vi "xc_umn_XPS_and_LockinControl_GPIB.vi"() -> ()   [LabVIEW 2013]
uses:
  <vilib>/Analysis/baseanly.llb/Mean (DBL).vi
  <vilib>/Utility/file.llb/Write To Spreadsheet File (DBL).vi
  <vilib>/Analysis/NI_AALBase.lvlib
panel:
  in  "?":string
  in  "?":T1(tab)
  out "Waveform Graph":dbl[](graph)=[0.0, -0.00745064, -0.0298025, -0.0149013, -0.00745064, 0.0, 0.00745064, 0.022351899999999997, 0.0149013, 0.00745064, -0.0298025, 0.0149013, 0.0, -0.0447037, -0.00745064, -0.00745064, 0.022351899999999997, 0.0, 0.0, -0.00745064, 0.037253100000000004, -0.00745064, -0.0298025, 0.0, -0.0149013, 0.0, 0.0, -0.0670557, -0.0149013, 0.0149013, 0.0149013, 0.0, 0.0, 0.0149013, 0.0, 0.0298025, -0.0447037, 0.00745064, -0.037253100000000004, -0.0149013, 0.00745064, 0.037253100000000004, 0.0149013, 0.0, -0.0298025, -0.0149013, 0.00745064, 0.0, -0.0447037, 0.00745064, 0.0149013, 0.022351899999999997, 0.0, -0.022351899999999997, 0.0, 0.037253100000000004, -0.0298025, -0.037253100000000004, -0.00745064, 0.0, -0.00745064, 0.0298025, 0.0149013, 0.0, -0.0298025, 0.0149013, -0.0298025, -0.0298025, -0.00745064, -0.0298025, -0.037253100000000004, -0.022351899999999997, 0.0, -0.0298025, -0.037253100000000004, 0.0149013, -0.00745064, -0.0149013, -0.00745064, 0.0, -0.0447037, 0.0149013, 0.0, -0.037253100000000004, -0.0149013, -0.0298025, -0.0447037, -0.022351899999999997, -0.022351899999999997, 0.0149013, -0.022351899999999997, 0.0, -0.022351899999999997, 0.022351899999999997, 0.0, 0.037253100000000004, -0.022351899999999997, 0.022351899999999997, -0.0298025, -0.022351899999999997]
  in  "Start Button":bool
  in  "quit Button":bool
  in  "save":bool
  out "Current Mean":dbl=-0.0275905 format="%#_10g"
  out "Current position":dbl=-9.999556
  in  "Range (in mm)":dbl=1.0
  in  "Increment (in mm)":dbl=0.01
  in  "Averages":u16=1
  in  "Start Position":dbl=-10.0
  in  "move":bool
  out "Compensation":dbl=1000000.0
  in  "Position":dbl
  in  "Left jog":bool
  in  "Jog step size (mm)":dbl=0.01
  in  "Right jog":bool
  out "Stage Position":dbl=1e-06
  in  "Move to Position Button":bool
  in  "Time Constant":u16(ring)=7 items=["10 us", "30 us", "100 us", "300 us", "1 ms", "3 ms", "10 ms", "30 ms", "100 ms", "300 ms", "1 s", "3 s", "10 s", "30 s", "100 s", "300 s", "1 ks", "3 ks", "10 ks", "30 ks"]
  in  "Sensitivity":u16(ring)=9 items=["2 nV/fA", "5 nV/fA", "10 nV/fA", "20 nV/fA", "50 nV/fA", "100 nV/fA", "200 nV/fA", "500 nV/fA", "1 uV/pA", "2 uV/pA", "5 uV/pA", "10 uV/pA", "20 uV/pA", "50 uV/pA", "100 uV/pA", "200 uV/pA", "500 uV/pA", "1 mV/nA", "2 mV/nA", "5 mV/nA", "10 mV/nA", "20 mV/nA", "50 mV/nA", "100 mV/nA", "200 mV/nA", "500 mV/nA", "1 V/uA"]
  in  "Input Configuration":u16(ring) items=["A", "A-B", "1 MOhm", "10 MOhm"]
  out "Sensitivity Compensation":dbl=1000000.0
  in  "Autophase":bool
  out "Scale Unit":string="uV"
  out "Lockin realtime output":dbl(knob)=-0.0275905 scale=-1.0..1.0
  out "Lockin error out":errorcluster={"status"=FALSE, "code"=1073676294, "source"="VISA Read in xc_umn_XPS_and_LockinControl.vi"}
  in  "Lockin error in":errorcluster
  out "Array":dbl[](array[numeric])=[0.0, -0.00745064, -0.0298025, -0.0149013, -0.00745064, 0.0, 0.00745064, 0.022351899999999997, 0.0149013, 0.00745064, -0.0298025, 0.0149013, 0.0, -0.0447037, -0.00745064, -0.00745064, 0.022351899999999997, 0.0, 0.0, -0.00745064, 0.037253100000000004, -0.00745064, -0.0298025, 0.0, -0.0149013, 0.0, 0.0, -0.0670557, -0.0149013, 0.0149013, 0.0149013, 0.0, 0.0, 0.0149013, 0.0, 0.0298025, -0.0447037, 0.00745064, -0.037253100000000004, -0.0149013, 0.00745064, 0.037253100000000004, 0.0149013, 0.0, -0.0298025, -0.0149013, 0.00745064, 0.0, -0.0447037, 0.00745064, 0.0149013, 0.022351899999999997, 0.0, -0.022351899999999997, 0.0, 0.037253100000000004, -0.0298025, -0.037253100000000004, -0.00745064, 0.0, -0.00745064, 0.0298025, 0.0149013, 0.0, -0.0298025, 0.0149013, -0.0298025, -0.0298025, -0.00745064, -0.0298025, -0.037253100000000004, -0.022351899999999997, 0.0, -0.0298025, -0.037253100000000004, 0.0149013, -0.00745064, -0.0149013, -0.00745064, 0.0, -0.0447037, 0.0149013, 0.0, -0.037253100000000004, -0.0149013, -0.0298025, -0.0447037, -0.022351899999999997, -0.022351899999999997, 0.0149013, -0.022351899999999997, 0.0, -0.022351899999999997, 0.022351899999999997, 0.0, 0.037253100000000004, -0.022351899999999997, 0.022351899999999997, -0.0298025, -0.022351899999999997]
  out "Array 2":dbl[](array[numeric])=[-9.989987, -9.979989, -9.969994, -9.959974, -9.949978, -9.939973, -9.929969, -9.919957, -9.909953, -9.899948, -9.889937, -9.879957, -9.869966, -9.85997, -9.849976, -9.839989, -9.82999, -9.819995, -9.809984, -9.799976, -9.789956, -9.77995, -9.769948, -9.759954, -9.749947, -9.739953, -9.729953, -9.719978, -9.70998, -9.699991, -9.689985, -9.679993, -9.669982, -9.660004, -9.649987, -9.639984, -9.629972, -9.619964, -9.609951, -9.59995, -9.58996, -9.579923, -9.569946, -9.559948, -9.549953, -9.539952, -9.529956, -9.519982, -9.509964, -9.499961, -9.489967, -9.479974, -9.469988, -9.459988, -9.449998, -9.439994, -9.429985, -9.419973, -9.409972, -9.399965, -9.389954, -9.37994, -9.369937, -9.35994, -9.349967, -9.339974, -9.330002, -9.319993, -9.309984, -9.299992, -9.289988, -9.279986, -9.269974, -9.259965, -9.249946, -9.239952, -9.229939, -9.219955, -9.209954, -9.199959, -9.189968, -9.179975, -9.169977, -9.159978, -9.149988, -9.139981, -9.129984, -9.119984, -9.109976, -9.099978, -9.089976, -9.07995, -9.069946, -9.059963, -9.049951, -9.039946, -9.029939, -9.019958, -9.009948, -8.999961]
  in  "Lockin GPIB Address":string
  in  "PI Stage Error":errorcluster
  out "PI Stage Error 2":errorcluster
  out "Identification":string="(c)2010 Physik Instrumente(PI) Karlsruhe, C-867.160,0,1.2.0.1"
  # "University of Minnesota Lockin Scan and Optimize\nVersion 2.0\n[XPS Controller; SR830 Lockin; RS232]"
  # "Lockin Output"
  # "Stage Controls"
  # "Lockin Controls"
  # "Lockin Communications"
  # "Stage Communications"
  # "Data Out"
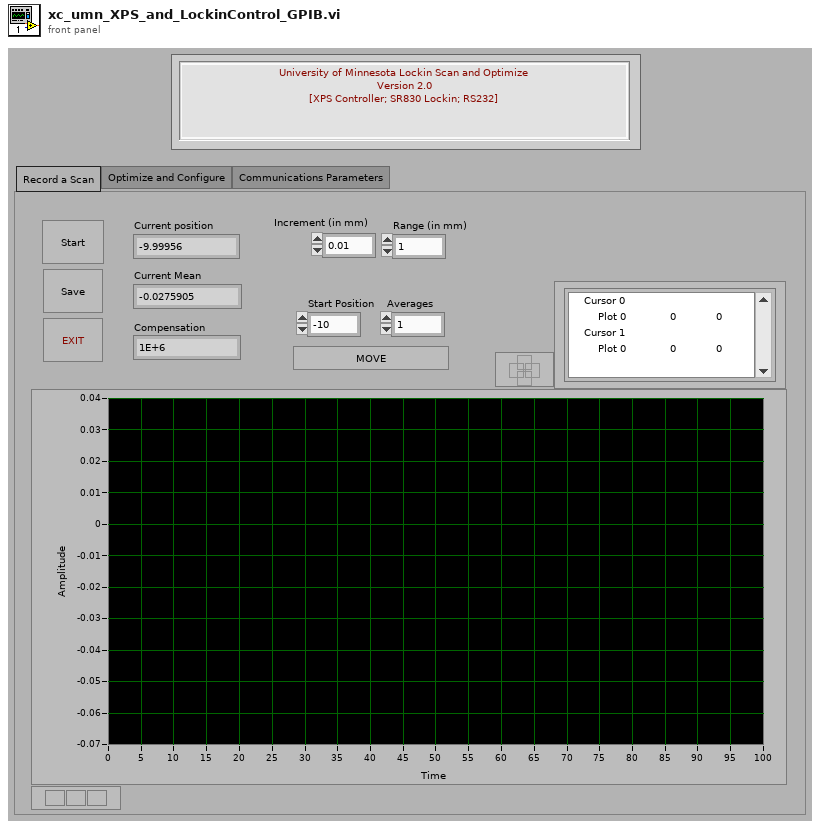
[diagram p1: front panel]
types:
  T1 = enum32{"Record a Scan", "Optimize and Configure", "Communications Parameters"}
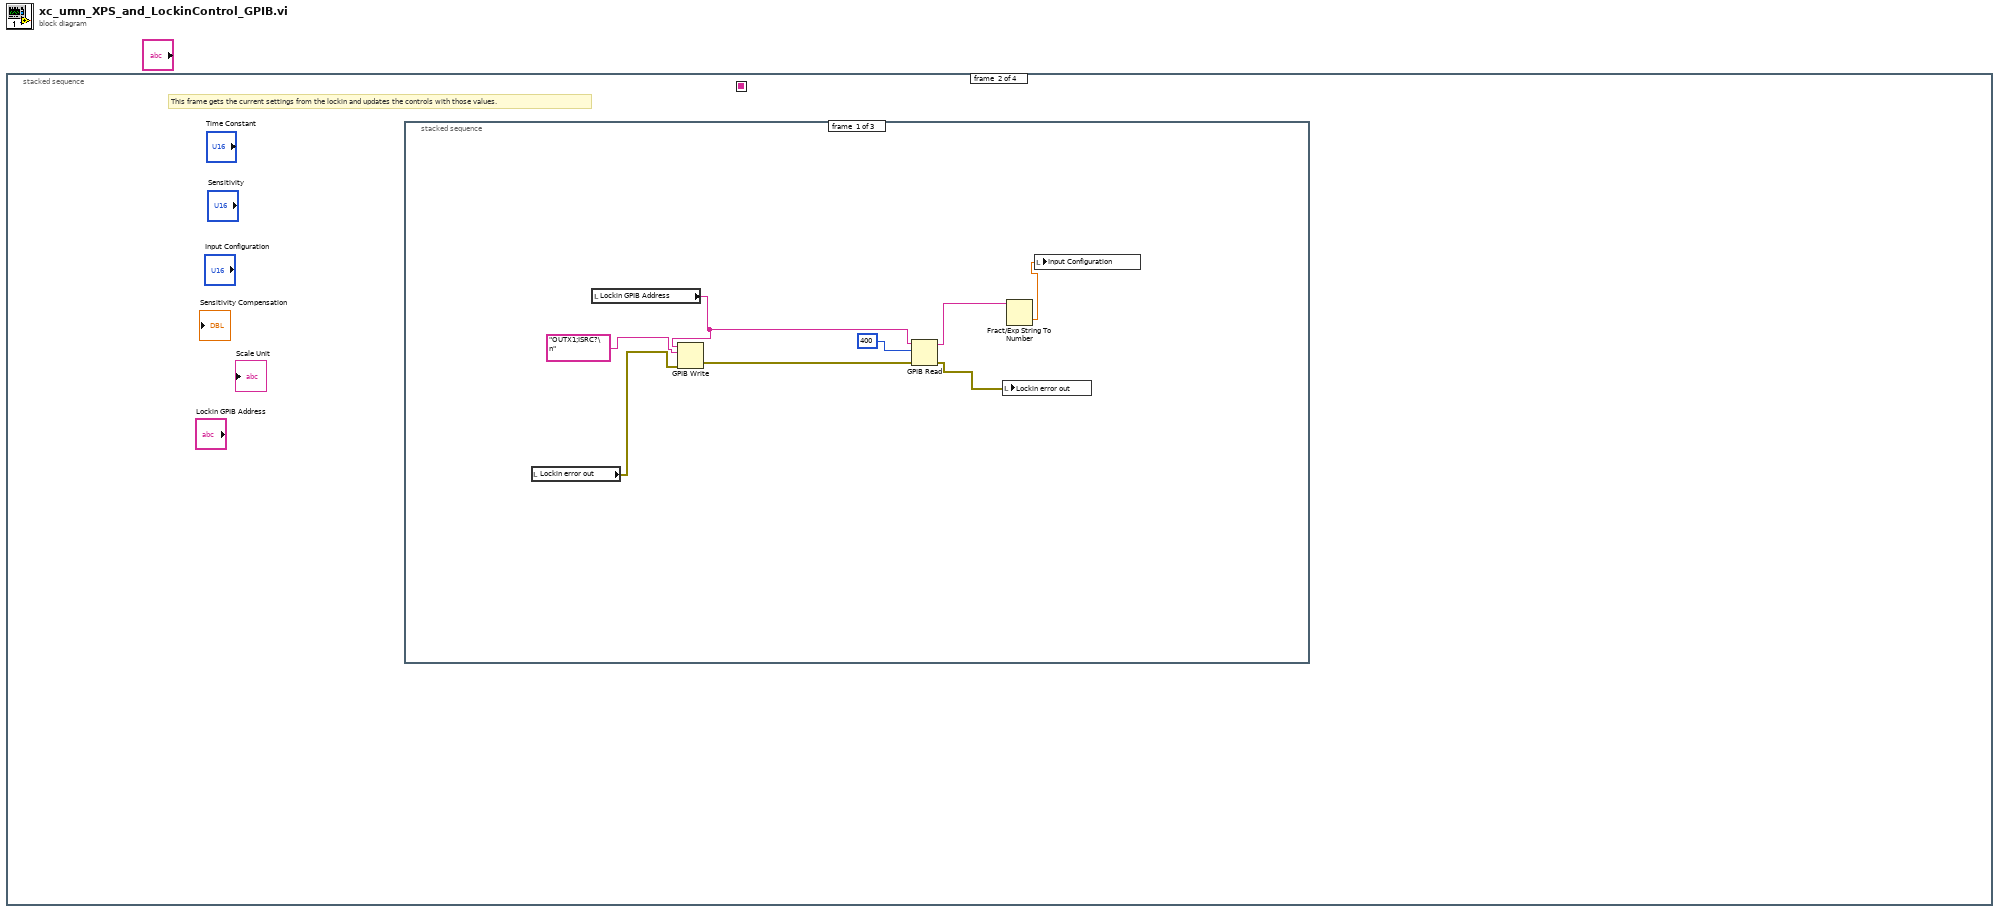
[diagram p0: block diagram]
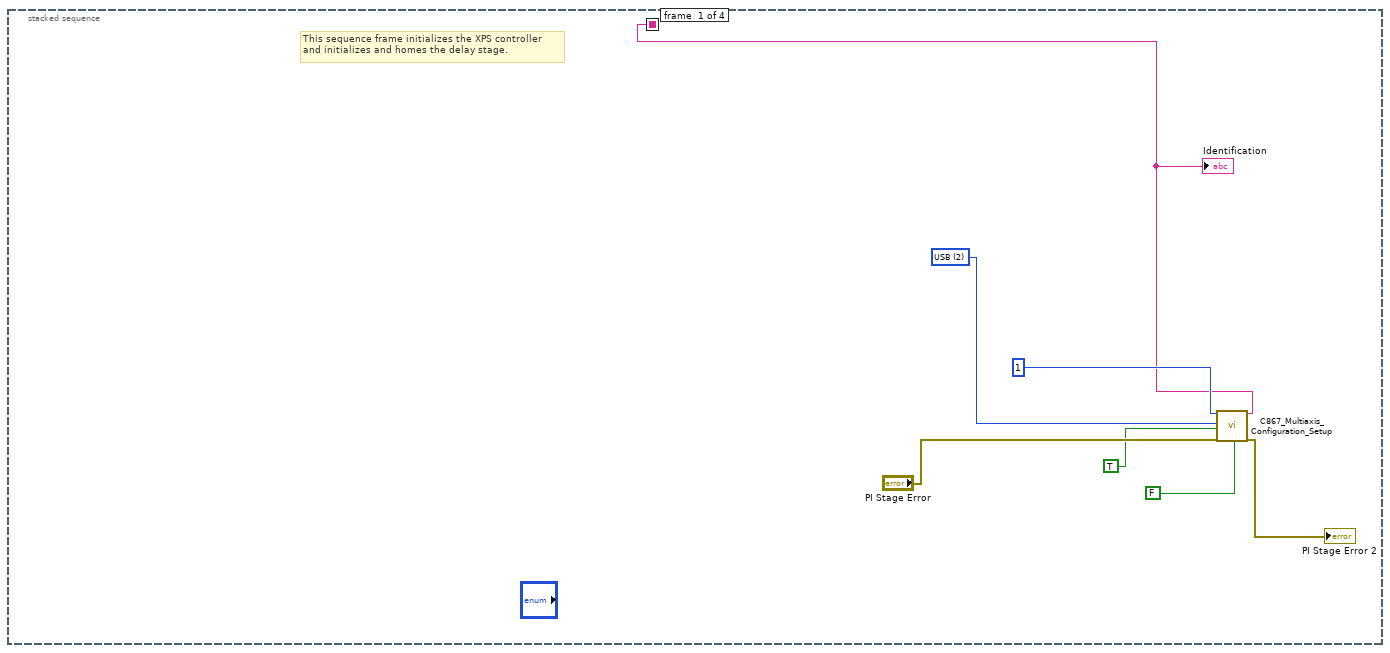
[diagram p2: hidden frame]
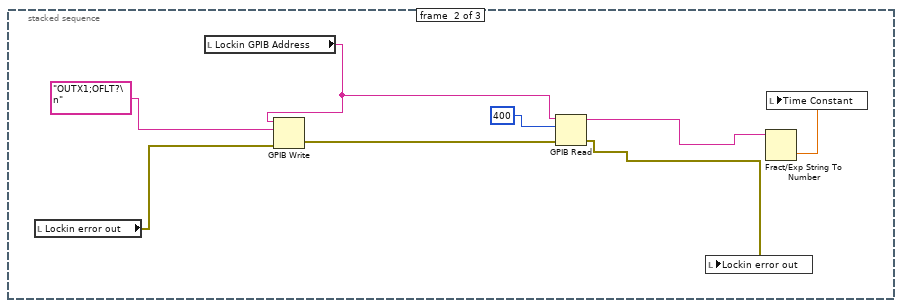
[diagram p3: hidden frame]
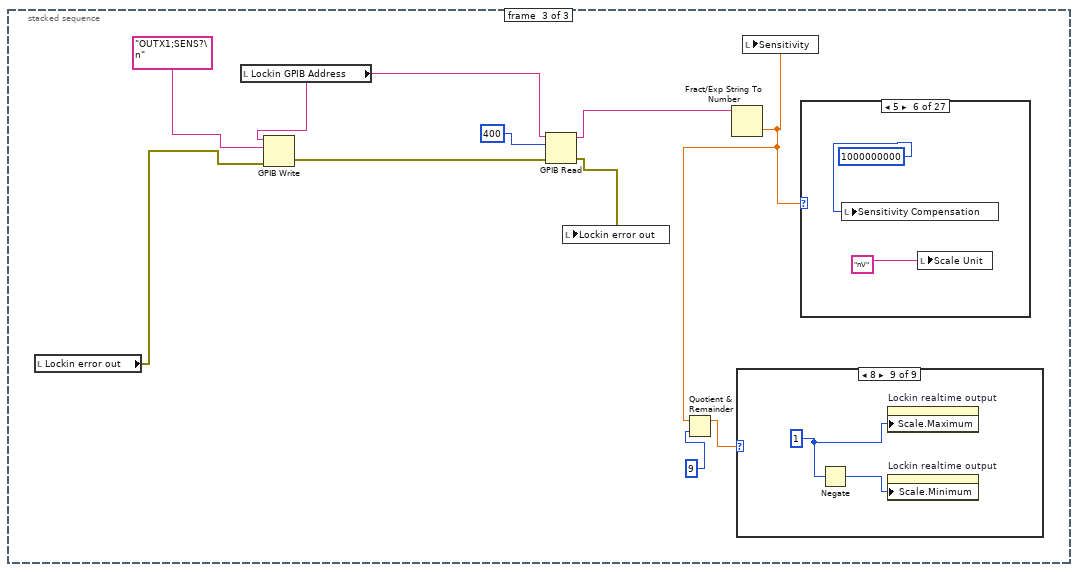
[diagram p4: hidden frame]
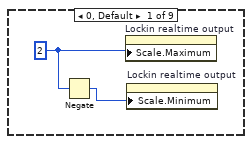
[diagram p5: hidden frame]
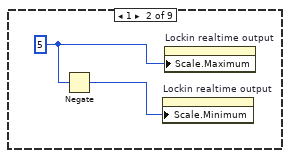
[diagram p6: hidden frame]
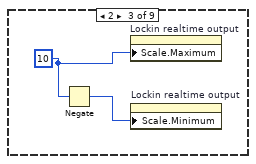
[diagram p7: hidden frame]
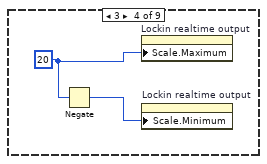
[diagram p8: hidden frame]
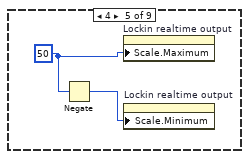
[diagram p9: hidden frame]
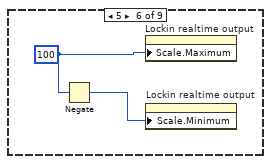
[diagram p10: hidden frame]
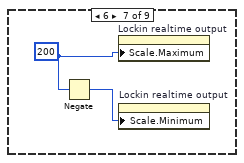
[diagram p11: hidden frame]
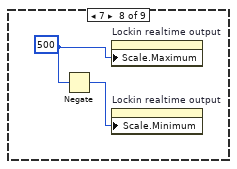
[diagram p12: hidden frame]
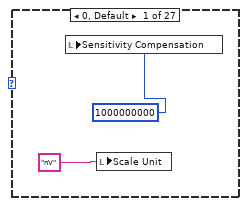
[diagram p13: hidden frame]
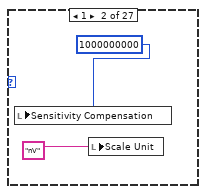
[diagram p14: hidden frame]
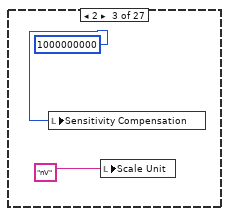
[diagram p15: hidden frame]
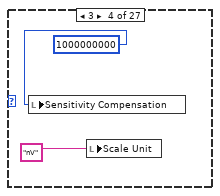
[diagram p16: hidden frame]
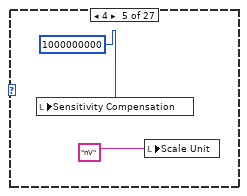
[diagram p17: hidden frame]
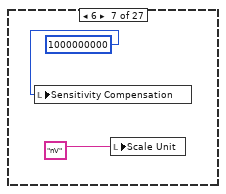
[diagram p18: hidden frame]
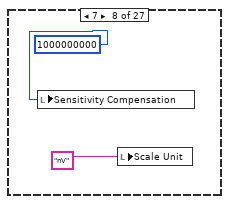
[diagram p19: hidden frame]
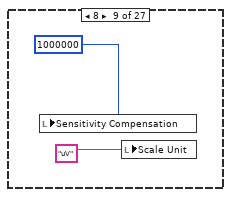
[diagram p20: hidden frame]
diagram:
  n1 = stacked-sequence {
    seq-local: [w1 _ _ _] -> [_ _ w109 _]
    frame #0 {
      w3 = u16 2 items=["RS232", "RS232 DaisyChain", "USB"] ("Interface")
      # "This sequence frame initializes the XPS controller \nand initializes and homes the delay stage."
      n2 = call "C867_Multiaxis_Configuration_Setup.vi"("System no."=1, "Interface"=w3, "All axes?"=TRUE, "error in"="PI Stage Error", "Switch servo on?"=FALSE) -> ("Identification"=w1:string, "error out"=→"PI Stage Error 2":errorcluster)  [unwired: 8 in, 5 out]
      "Identification" <- w1
    }
    frame #1 {
      # "This frame gets the current settings from the lockin and updates the controls with those values."
      n3 = stacked-sequence {
        frame #0 {
          n4 = local read "Lockin error out"() -> (w11:errorcluster)
          n5 = local read "Lockin GPIB Address"() -> (w12:string)
          n6 = GPIB Write(0:w12, 1:"OUTX1;ISRC?\n", 3:w11) -> (6:w14:errorcluster)  [unwired: 2 in, 1 out]
          n7 = GPIB Read(0:w12, 1:400, 3:w14) -> (5:w8:string, 7:w9:errorcluster)  [unwired: 2 in, 1 out]
          n8 = local write "Lockin error out"(w9) -> ()
          n9 = Fract/Exp String To Number(string=w8) -> (number=w15:dbl)  [unwired: 3 in, 1 out]
          n10 = local write "Input Configuration"(w15) -> ()
        }
        frame #1 {
          n11 = local read "Lockin error out"() -> (w16:errorcluster)
          n12 = local read "Lockin GPIB Address"() -> (w18:string)
          n13 = GPIB Write(0:w18, 1:"OUTX1;OFLT?\n", 3:w16) -> (6:w22:errorcluster)  [unwired: 2 in, 1 out]
          n14 = GPIB Read(0:w18, 1:400, 3:w22) -> (5:w19:string, 7:w20:errorcluster)  [unwired: 2 in, 1 out]
          n15 = local write "Lockin error out"(w20) -> ()
          n16 = Fract/Exp String To Number(string=w19) -> (number=w23:dbl)  [unwired: 3 in, 1 out]
          n17 = local write "Time Constant"(w23) -> ()
        }
        frame #2 {
          n18 = local read "Lockin error out"() -> (w29:errorcluster)
          n19 = local read "Lockin GPIB Address"() -> (w24:string)
          n20 = GPIB Write(0:w24, 1:"OUTX1;SENS?\n", 3:w29) -> (6:w26:errorcluster)  [unwired: 2 in, 1 out]
          n21 = GPIB Read(0:w24, 1:400, 3:w26) -> (5:w28:string, 7:w27:errorcluster)  [unwired: 2 in, 1 out]
          n22 = local write "Lockin error out"(w27) -> ()
          n23 = Fract/Exp String To Number(string=w28) -> (number=w31:dbl)  [unwired: 3 in, 1 out]
          n24 = Quotient & Remainder(x=w31, y=9) -> (x-y*floor(x/y)=w32:dbl)  [unwired: 1 out]
          n25 = case shown="8" w32 {
            frame 0, Default {
              w35 = 2
              n26 = Negate(x=w35) -> (-x=w34:i32)
              n27 = property on="Lockin realtime output" class="Knob (strict)"("Scale.Maximum"=w35) -> ()  [unwired: 2 in, 2 out]
              n28 = property on="Lockin realtime output" class="Knob (strict)"("Scale.Minimum"=w34) -> ()  [unwired: 2 in, 2 out]
            }
            frame 1 {
              w37 = 5
              n29 = Negate(x=w37) -> (-x=w36:i32)
              n30 = property on="Lockin realtime output" class="Knob (strict)"("Scale.Minimum"=w36) -> ()  [unwired: 2 in, 2 out]
              n31 = property on="Lockin realtime output" class="Knob (strict)"("Scale.Maximum"=w37) -> ()  [unwired: 2 in, 2 out]
            }
            frame 2 {
              w38 = 10
              n32 = Negate(x=w38) -> (-x=w39:i32)
              n33 = property on="Lockin realtime output" class="Knob (strict)"("Scale.Maximum"=w38) -> ()  [unwired: 2 in, 2 out]
              n34 = property on="Lockin realtime output" class="Knob (strict)"("Scale.Minimum"=w39) -> ()  [unwired: 2 in, 2 out]
            }
            frame 3 {
              w40 = 20
              n35 = Negate(x=w40) -> (-x=w41:i32)
              n36 = property on="Lockin realtime output" class="Knob (strict)"("Scale.Maximum"=w40) -> ()  [unwired: 2 in, 2 out]
              n37 = property on="Lockin realtime output" class="Knob (strict)"("Scale.Minimum"=w41) -> ()  [unwired: 2 in, 2 out]
            }
            frame 4 {
              w42 = 50
              n38 = Negate(x=w42) -> (-x=w43:i32)
              n39 = property on="Lockin realtime output" class="Knob (strict)"("Scale.Maximum"=w42) -> ()  [unwired: 2 in, 2 out]
              n40 = property on="Lockin realtime output" class="Knob (strict)"("Scale.Minimum"=w43) -> ()  [unwired: 2 in, 2 out]
            }
            frame 5 {
              w44 = 100
              n41 = Negate(x=w44) -> (-x=w45:i32)
              n42 = property on="Lockin realtime output" class="Knob (strict)"("Scale.Maximum"=w44) -> ()  [unwired: 2 in, 2 out]
              n43 = property on="Lockin realtime output" class="Knob (strict)"("Scale.Minimum"=w45) -> ()  [unwired: 2 in, 2 out]
            }
            frame 6 {
              w46 = 200
              n44 = Negate(x=w46) -> (-x=w47:i32)
              n45 = property on="Lockin realtime output" class="Knob (strict)"("Scale.Maximum"=w46) -> ()  [unwired: 2 in, 2 out]
              n46 = property on="Lockin realtime output" class="Knob (strict)"("Scale.Minimum"=w47) -> ()  [unwired: 2 in, 2 out]
            }
            frame 7 {
              w49 = 500
              n47 = Negate(x=w49) -> (-x=w48:i32)
              n48 = property on="Lockin realtime output" class="Knob (strict)"("Scale.Maximum"=w49) -> ()  [unwired: 2 in, 2 out]
              n49 = property on="Lockin realtime output" class="Knob (strict)"("Scale.Minimum"=w48) -> ()  [unwired: 2 in, 2 out]
            }
            frame 8 {
              w50 = 1
              n50 = Negate(x=w50) -> (-x=w51:i32)
              n51 = property on="Lockin realtime output" class="Knob (strict)"("Scale.Maximum"=w50) -> ()  [unwired: 2 in, 2 out]
              n52 = property on="Lockin realtime output" class="Knob (strict)"("Scale.Minimum"=w51) -> ()  [unwired: 2 in, 2 out]
            }
          }
          n53 = local write "Sensitivity"(w31) -> ()
          n54 = case shown="5" w31 {
            frame 0, Default {
              n55 = local write "Sensitivity Compensation"(1000000000) -> ()
              n56 = local write "Scale Unit"("nV") -> ()
            }
            frame 1 {
              n57 = local write "Sensitivity Compensation"(1000000000) -> ()
              n58 = local write "Scale Unit"("nV") -> ()
            }
            frame 2 {
              n59 = local write "Sensitivity Compensation"(1000000000) -> ()
              n60 = local write "Scale Unit"("nV") -> ()
            }
            frame 3 {
              n61 = local write "Sensitivity Compensation"(1000000000) -> ()
              n62 = local write "Scale Unit"("nV") -> ()
            }
            frame 4 {
              n63 = local write "Sensitivity Compensation"(1000000000) -> ()
              n64 = local write "Scale Unit"("nV") -> ()
            }
            frame 5 {
              n65 = local write "Sensitivity Compensation"(1000000000) -> ()
              n66 = local write "Scale Unit"("nV") -> ()
            }
            frame 6 {
              n67 = local write "Sensitivity Compensation"(1000000000) -> ()
              n68 = local write "Scale Unit"("nV") -> ()
            }
            frame 7 {
              n69 = local write "Sensitivity Compensation"(1000000000) -> ()
              n70 = local write "Scale Unit"("nV") -> ()
            }
            frame 8 {
              n71 = local write "Sensitivity Compensation"(1000000) -> ()
              n72 = local write "Scale Unit"("uV") -> ()
            }
            frame 9 {
              n73 = local write "Sensitivity Compensation"(1000000) -> ()
              n74 = local write "Scale Unit"("uV") -> ()
            }
            frame 10 {
              n75 = local write "Sensitivity Compensation"(1000000) -> ()
              n76 = local write "Scale Unit"("uV") -> ()
            }
            frame 11 {
              n77 = local write "Sensitivity Compensation"(1000000) -> ()
              n78 = local write "Scale Unit"("uV") -> ()
            }
            frame 12 {
              n79 = local write "Sensitivity Compensation"(1000000) -> ()
              n80 = local write "Scale Unit"("uV") -> ()
            }
            frame 13 {
              n81 = local write "Sensitivity Compensation"(1000000) -> ()
              n82 = local write "Scale Unit"("uV") -> ()
            }
            frame 14 {
              n83 = local write "Sensitivity Compensation"(1000000) -> ()
              n84 = local write "Scale Unit"("uV") -> ()
            }
            frame 15 {
              n85 = local write "Sensitivity Compensation"(1000000) -> ()
              n86 = local write "Scale Unit"("uV") -> ()
            }
            frame 16 {
              n87 = local write "Sensitivity Compensation"(1000000) -> ()
              n88 = local write "Scale Unit"("uV") -> ()
            }
            frame 17 {
              n89 = local write "Sensitivity Compensation"(1000) -> ()
              n90 = local write "Scale Unit"("mV") -> ()
            }
            frame 18 {
              n91 = local write "Sensitivity Compensation"(1000) -> ()
              n92 = local write "Scale Unit"("mV") -> ()
            }
            frame 19 {
              n93 = local write "Sensitivity Compensation"(1000) -> ()
              n94 = local write "Scale Unit"("mV") -> ()
            }
            frame 20 {
              n95 = local write "Sensitivity Compensation"(1000) -> ()
              n96 = local write "Scale Unit"("mV") -> ()
            }
            frame 21 {
              n97 = local write "Sensitivity Compensation"(1000) -> ()
              n98 = local write "Scale Unit"("mV") -> ()
            }
            frame 22 {
              n99 = local write "Sensitivity Compensation"(1000) -> ()
              n100 = local write "Scale Unit"("mV") -> ()
            }
            frame 23 {
              n101 = local write "Sensitivity Compensation"(1000) -> ()
              n102 = local write "Scale Unit"("mV") -> ()
            }
            frame 24 {
              n103 = local write "Sensitivity Compensation"(1000) -> ()
              n104 = local write "Scale Unit"("mV") -> ()
            }
            frame 25 {
              n105 = local write "Sensitivity Compensation"(1000) -> ()
              n106 = local write "Scale Unit"("mV") -> ()
            }
            frame 26 {
              n107 = local write "Sensitivity Compensation"(1) -> ()
              n108 = local write "Scale Unit"("V") -> ()
            }
          }
        }
      }
    }
    frame #2 {
      n109 = local read "Input Configuration"() -> (w108:u16)
      n110 = local read "Time Constant"() -> (w107:u16)
      n111 = local read "Sensitivity"() -> (w106:u16)
      n112 = while {
        tunnel: w109 -> [w116]
        shift-right: [w114] -> _
        shift-left: w108 -> [w115]
        shift-right: [w112] -> _
        shift-left: w107 -> [w113]
        shift-right: [w110] -> _
        shift-left: w106 -> [w111]
        stop <- "quit Button" stop-if-true
        # "This panel does the scanning and lockin readout (when not scanning)"
        n113 = stacked-sequence {
          tunnel: w116 -> [w118 w175 w191]
          tunnel: w115 -> [_ _ w189]
          tunnel: [_ _ w188] -> w114
          tunnel: w113 -> [_ _ w187]
          tunnel: [_ _ w186] -> w112
          tunnel: w111 -> [_ _ w185]
          tunnel: [_ _ w184] -> w110
          frame #0 {
            n114 = case shown="True" "Start Button" {
              tunnel: w118 -> [_ w120]
              frame False {
              }
              frame True {
                n115 = stacked-sequence {
                  tunnel: w120 -> [w121 _ _]
                  frame #0 {
                    n116 = Initialize Array(0) -> (w124:i32[])  [unwired: 1 in]
                    n117 = Divide(x="Range (in mm)", y="Increment (in mm)") -> (x/y=w127:dbl)
                    n118 = To Word Integer(number=w127) -> (16bit integer=w126:i16)
                    n119 = for {
                      N: w126 -> [_]
                      shift-right: [w133] -> _
                      shift-left: w124 -> [w134]
                      tunnel: [w132] -> w123 mode=indexing
                      tunnel: [w131] -> w122 mode=indexing
                      tunnel: w121 -> [w130]
                      i -> [w136]
                      n120 = local read "Start Button"() -> (w137:bool)
                      n121 = case shown="True" w137 {
                        tunnel: w136 -> [_ w146]
                        tunnel: [w138 w142] -> w135
                        tunnel: [w138 w142] -> w132
                        tunnel: [w138 w144] -> w131
                        tunnel: w130 -> [_ w141]
                        frame False {
                          w138 = 0
                          n122 = Build Array(0) -> ()  [unwired: 1 out]
                        }
                        frame True {
                          n123 = stacked-sequence {
                            tunnel: w146 -> [w151 _]
                            tunnel: [_ w157] -> w145
                            tunnel: [w149 _] -> w144
                            tunnel: w141 -> [_ _]
                            frame #0 {
                              n124 = local read "Increment (in mm)"() -> (w153:dbl)
                              n125 = local read "PI Stage Error"() -> (w148:errorcluster)
                              n126 = Add(x=w151, y=1) -> (x+y=w154:i32)
                              n127 = Multiply(x=w153, y=w154) -> (x*y=w155:dbl)
                              n128 = Add(x="Start Position", y=w155) -> (x+y=w150:dbl)
                              n129 = call "movePI.vi"("PI Stage Error"=w148, "move to position"=w150) -> ("final position"=w149:dbl, "PI Stage Error 2"=w147:errorcluster)
                              "Current position" <- w149
                              n130 = local write "PI Stage Error"(w147) -> ()
                            }
                            frame #1 {
                              n131 = for {
                                N: "Averages" -> [_]
                                tunnel: [w166] -> w157 mode=indexing
                                n132 = local read "Lockin GPIB Address"() -> (w160:string)
                                n133 = GPIB Write(0:w160, 1:"OUTX1;OUTP?1\n" ("string to write"), 3:"Lockin error in") -> (6:w165:errorcluster)  [unwired: 2 in, 1 out]
                                n134 = GPIB Read(0:w160, 1:400, 3:w165) -> (5:w159:string, 7:→"Lockin error out":errorcluster)  [unwired: 2 in, 1 out]
                                n135 = Fract/Exp String To Number(string=w159) -> (number=w166:dbl)  [unwired: 3 in, 1 out]
                              }
                            }
                          }
                          n136 = local read "Sensitivity Compensation"() -> (w140:dbl)
                          "Compensation" <- w140
                          n137 = call-poly <vilib>:"Mean.vi"("X"=w145) -> ("mean"=w143:dbl)  [unwired: 1 out]
                          n138 = Multiply(x=w143, y=w140) -> (x*y=w142:dbl)
                          "Current Mean" <- w142
                        }
                      }
                      n139 = Build Array (concatenate)(w134, w135) -> (w133:dbl[])
                      "Waveform Graph" <- w133
                    }
                    "Array" <- w123
                    "Array 2" <- w122
                  }
                  frame #1 {
                    n140 = case shown="True" "save" {
                      frame False {
                        n141 = local write "save"(FALSE) -> ()
                      }
                      frame True {
                        n142 = local read "Array 2"() -> (w169:dbl[])
                        n143 = local read "Array"() -> (w170:dbl[])
                        n144 = Build Array(w170, w169) -> (w172:dbl[][])
                        n145 = Transpose 2D Array(2D array=w172) -> (transposed array=w171:dbl[][])
                        n146 = call-poly <vilib>:"Write To Spreadsheet File.vi"("format (%.3f)"="%.8f", "2D data"=w171) -> ()  [unwired: 6 in, 1 out]
                      }
                    }
                  }
                  frame #2 {
                    n147 = local write "Start Button"(FALSE) -> ()
                  }
                }
              }
            }
          }
          frame #1 {
            # "This is the move button for starting a scan"
            n148 = case shown="True" "move" {
              tunnel: w175 -> [_ w177]
              frame False {
              }
              frame True {
                n149 = stacked-sequence {
                  tunnel: w177 -> [_ _ _]
                  frame #0 {
                    n150 = local read "PI Stage Error 2"() -> (w180:errorcluster)
                    n151 = local read "Start Position"() -> (w181:dbl)
                    n152 = call "movePI.vi"("PI Stage Error"=w180, "move to position"=w181) -> ("final position"=w179:dbl, "PI Stage Error 2"=w178:errorcluster)
                    n153 = local write "Current position"(w179) -> ()
                    n154 = local write "PI Stage Error 2"(w178) -> ()
                  }
                  frame #1 {
                    n155 = Wait Until Next ms Multiple(millisecond multiple=u32 50) -> ()  [unwired: 1 out]
                  }
                  frame #2 {
                    n156 = local write "move"(FALSE) -> ()
                  }
                }
              }
            }
          }
          frame #2 {
            # "This loop does the realtime lockin updating and readout"
            # "These are all the rest of the buttons"
            n157 = local read "Jog step size (mm)"() -> (w201:dbl)
            n158 = stacked-sequence {
              tunnel: w189 -> [w212 _ _ _]
              tunnel: [w210 _ _ _] -> w188
              tunnel: w187 -> [_ w226 _ _]
              tunnel: [_ w223 _ _] -> w186
              tunnel: w185 -> [_ _ w239 _]
              tunnel: [_ _ w236 _] -> w184
              frame #0 {
                n159 = local read "Input Configuration"() -> (w213:u16)
                n160 = Not Equal?(x=w213, y=w212) -> (x != y?=w211:bool)
                n161 = case shown="True" w211 {
                  tunnel: [w214 w222] -> w210
                  frame False {
                    n162 = local read "Input Configuration"() -> (w214:u16)
                  }
                  frame True {
                    n163 = local read "Lockin GPIB Address"() -> (w216:string)
                    n164 = local read "Lockin error out"() -> (w218:errorcluster)
                    n165 = local read "Input Configuration"() -> (w222:u16)
                    n166 = Number To Decimal String(number=w222) -> (decimal integer string=w221:string)  [unwired: 1 in]
                    n167 = Concatenate Strings("OUTX0;ISRC", w221, "\r") -> (w215:string)
                    n168 = GPIB Write(0:w216, 1:w215, 3:w218) -> (6:w217:errorcluster)  [unwired: 2 in, 1 out]
                    n169 = local write "Lockin error out"(w217) -> ()
                  }
                }
              }
              frame #1 {
                n170 = local read "Time Constant"() -> (w225:u16)
                n171 = Not Equal?(x=w225, y=w226) -> (x != y?=w224:bool)
                n172 = case shown="True" w224 {
                  tunnel: [w227 w235] -> w223
                  frame False {
                    n173 = local read "Time Constant"() -> (w227:u16)
                  }
                  frame True {
                    n174 = local read "Lockin GPIB Address"() -> (w231:string)
                    n175 = local read "Lockin error in"() -> (w229:errorcluster)
                    n176 = local read "Time Constant"() -> (w235:u16)
                    n177 = Number To Decimal String(number=w235) -> (decimal integer string=w234:string)  [unwired: 1 in]
                    n178 = Concatenate Strings("OUTX0;OFLT", w234, "\r") -> (w230:string)
                    n179 = GPIB Write(0:w231, 1:w230, 3:w229) -> (6:w228:errorcluster)  [unwired: 2 in, 1 out]
                    n180 = local write "Lockin error out"(w228) -> ()
                  }
                }
              }
              frame #2 {
                n181 = local read "Sensitivity"() -> (w238:u16)
                n182 = Not Equal?(x=w238, y=w239) -> (x != y?=w237:bool)
                n183 = case shown="True" w237 {
                  tunnel: [w240 w245] -> w236
                  frame False {
                    n184 = local read "Sensitivity"() -> (w240:u16)
                  }
                  frame True {
                    n185 = local read "Lockin GPIB Address"() -> (w242:string)
                    n186 = local read "Lockin error out"() -> (w244:errorcluster)
                    n187 = local read "Sensitivity"() -> (w245:u16)
                    n188 = Number To Decimal String(number=w245) -> (decimal integer string=w250:string)  [unwired: 1 in]
                    n189 = Concatenate Strings("OUTX0;SENS", w250, "\r") -> (w241:string)
                    n190 = GPIB Write(0:w242, 1:w241, 3:w244) -> (6:w243:errorcluster)  [unwired: 2 in, 1 out]
                    n191 = local write "Lockin error out"(w243) -> ()
                    n192 = case shown="5" w245 {
                      frame 0, Default {
                        n193 = local write "Sensitivity Compensation"(1000000000) -> ()
                        n194 = local write "Scale Unit"("nV") -> ()
                      }
                      frame 1 {
                        n195 = local write "Sensitivity Compensation"(1000000000) -> ()
                        n196 = local write "Scale Unit"("nV") -> ()
                      }
                      frame 2 {
                        n197 = local write "Sensitivity Compensation"(1000000000) -> ()
                        n198 = local write "Scale Unit"("nV") -> ()
                      }
                      frame 3 {
                        n199 = local write "Sensitivity Compensation"(1000000000) -> ()
                        n200 = local write "Scale Unit"("nV") -> ()
                      }
                      frame 4 {
                        n201 = local write "Sensitivity Compensation"(1000000000) -> ()
                        n202 = local write "Scale Unit"("nV") -> ()
                      }
                      frame 5 {
                        n203 = local write "Sensitivity Compensation"(1000000000) -> ()
                        n204 = local write "Scale Unit"("nV") -> ()
                      }
                      frame 6 {
                        n205 = local write "Sensitivity Compensation"(1000000000) -> ()
                        n206 = local write "Scale Unit"("nV") -> ()
                      }
                      frame 7 {
                        n207 = local write "Sensitivity Compensation"(1000000000) -> ()
                        n208 = local write "Scale Unit"("nV") -> ()
                      }
                      frame 8 {
                        n209 = local write "Sensitivity Compensation"(1000000) -> ()
                        n210 = local write "Scale Unit"("uV") -> ()
                      }
                      frame 9 {
                        n211 = local write "Sensitivity Compensation"(1000000) -> ()
                        n212 = local write "Scale Unit"("uV") -> ()
                      }
                      frame 10 {
                        n213 = local write "Sensitivity Compensation"(1000000) -> ()
                        n214 = local write "Scale Unit"("uV") -> ()
                      }
                      frame 11 {
                        n215 = local write "Sensitivity Compensation"(1000000) -> ()
                        n216 = local write "Scale Unit"("uV") -> ()
                      }
                      frame 12 {
                        n217 = local write "Sensitivity Compensation"(1000000) -> ()
                        n218 = local write "Scale Unit"("uV") -> ()
                      }
                      frame 13 {
                        n219 = local write "Sensitivity Compensation"(1000000) -> ()
                        n220 = local write "Scale Unit"("uV") -> ()
                      }
                      frame 14 {
                        n221 = local write "Sensitivity Compensation"(1000000) -> ()
                        n222 = local write "Scale Unit"("uV") -> ()
                      }
                      frame 15 {
                        n223 = local write "Sensitivity Compensation"(1000000) -> ()
                        n224 = local write "Scale Unit"("uV") -> ()
                      }
                      frame 16 {
                        n225 = local write "Sensitivity Compensation"(1000000) -> ()
                        n226 = local write "Scale Unit"("uV") -> ()
                      }
                      frame 17 {
                        n227 = local write "Sensitivity Compensation"(1000) -> ()
                        n228 = local write "Scale Unit"("mV") -> ()
                      }
                      frame 18 {
                        n229 = local write "Sensitivity Compensation"(1000) -> ()
                        n230 = local write "Scale Unit"("mV") -> ()
                      }
                      frame 19 {
                        n231 = local write "Sensitivity Compensation"(1000) -> ()
                        n232 = local write "Scale Unit"("mV") -> ()
                      }
                      frame 20 {
                        n233 = local write "Sensitivity Compensation"(1000) -> ()
                        n234 = local write "Scale Unit"("mV") -> ()
                      }
                      frame 21 {
                        n235 = local write "Sensitivity Compensation"(1000) -> ()
                        n236 = local write "Scale Unit"("mV") -> ()
                      }
                      frame 22 {
                        n237 = local write "Sensitivity Compensation"(1000) -> ()
                        n238 = local write "Scale Unit"("mV") -> ()
                      }
                      frame 23 {
                        n239 = local write "Sensitivity Compensation"(1000) -> ()
                        n240 = local write "Scale Unit"("mV") -> ()
                      }
                      frame 24 {
                        n241 = local write "Sensitivity Compensation"(1000) -> ()
                        n242 = local write "Scale Unit"("mV") -> ()
                      }
                      frame 25 {
                        n243 = local write "Sensitivity Compensation"(1000) -> ()
                        n244 = local write "Scale Unit"("mV") -> ()
                      }
                      frame 26 {
                        n245 = local write "Sensitivity Compensation"(1) -> ()
                        n246 = local write "Scale Unit"("V") -> ()
                      }
                    }
                    n247 = Quotient & Remainder(x=w245, y=9) -> (x-y*floor(x/y)=w247:i32)  [unwired: 1 out]
                    n248 = case shown="8" w247 {
                      frame 0, Default {
                        w252 = 2
                        n249 = Negate(x=w252) -> (-x=w251:i32)
                        n250 = property on="Lockin realtime output" class="Knob (strict)"("Scale.Maximum"=w252) -> ()  [unwired: 2 in, 2 out]
                        n251 = property on="Lockin realtime output" class="Knob (strict)"("Scale.Minimum"=w251) -> ()  [unwired: 2 in, 2 out]
                      }
                      frame 1 {
                        w254 = 5
                        n252 = Negate(x=w254) -> (-x=w253:i32)
                        n253 = property on="Lockin realtime output" class="Knob (strict)"("Scale.Minimum"=w253) -> ()  [unwired: 2 in, 2 out]
                        n254 = property on="Lockin realtime output" class="Knob (strict)"("Scale.Maximum"=w254) -> ()  [unwired: 2 in, 2 out]
                      }
                      frame 2 {
                        w255 = 10
                        n255 = Negate(x=w255) -> (-x=w256:i32)
                        n256 = property on="Lockin realtime output" class="Knob (strict)"("Scale.Maximum"=w255) -> ()  [unwired: 2 in, 2 out]
                        n257 = property on="Lockin realtime output" class="Knob (strict)"("Scale.Minimum"=w256) -> ()  [unwired: 2 in, 2 out]
                      }
                      frame 3 {
                        w257 = 20
                        n258 = Negate(x=w257) -> (-x=w258:i32)
                        n259 = property on="Lockin realtime output" class="Knob (strict)"("Scale.Maximum"=w257) -> ()  [unwired: 2 in, 2 out]
                        n260 = property on="Lockin realtime output" class="Knob (strict)"("Scale.Minimum"=w258) -> ()  [unwired: 2 in, 2 out]
                      }
                      frame 4 {
                        w259 = 50
                        n261 = Negate(x=w259) -> (-x=w260:i32)
                        n262 = property on="Lockin realtime output" class="Knob (strict)"("Scale.Maximum"=w259) -> ()  [unwired: 2 in, 2 out]
                        n263 = property on="Lockin realtime output" class="Knob (strict)"("Scale.Minimum"=w260) -> ()  [unwired: 2 in, 2 out]
                      }
                      frame 5 {
                        w261 = 100
                        n264 = Negate(x=w261) -> (-x=w262:i32)
                        n265 = property on="Lockin realtime output" class="Knob (strict)"("Scale.Maximum"=w261) -> ()  [unwired: 2 in, 2 out]
                        n266 = property on="Lockin realtime output" class="Knob (strict)"("Scale.Minimum"=w262) -> ()  [unwired: 2 in, 2 out]
                      }
                      frame 6 {
                        w263 = 200
                        n267 = Negate(x=w263) -> (-x=w264:i32)
                        n268 = property on="Lockin realtime output" class="Knob (strict)"("Scale.Maximum"=w263) -> ()  [unwired: 2 in, 2 out]
                        n269 = property on="Lockin realtime output" class="Knob (strict)"("Scale.Minimum"=w264) -> ()  [unwired: 2 in, 2 out]
                      }
                      frame 7 {
                        w266 = 500
                        n270 = Negate(x=w266) -> (-x=w265:i32)
                        n271 = property on="Lockin realtime output" class="Knob (strict)"("Scale.Maximum"=w266) -> ()  [unwired: 2 in, 2 out]
                        n272 = property on="Lockin realtime output" class="Knob (strict)"("Scale.Minimum"=w265) -> ()  [unwired: 2 in, 2 out]
                      }
                      frame 8 {
                        w267 = 1
                        n273 = Negate(x=w267) -> (-x=w268:i32)
                        n274 = property on="Lockin realtime output" class="Knob (strict)"("Scale.Maximum"=w267) -> ()  [unwired: 2 in, 2 out]
                        n275 = property on="Lockin realtime output" class="Knob (strict)"("Scale.Minimum"=w268) -> ()  [unwired: 2 in, 2 out]
                      }
                    }
                  }
                }
              }
              frame #3 {
                n276 = local read "Averages"() -> (w327:u16)
                n277 = for {
                  N: w327 -> [_]
                  tunnel: [w335] -> w326 mode=indexing
                  n278 = local read "PI Stage Error 2"() -> (w331:errorcluster)
                  n279 = local read "Lockin GPIB Address"() -> (w328:string)
                  n280 = GPIB Write(0:w328, 1:"OUTX1;OUTP?1\n" ("string to write"), 3:w331) -> (6:w334:errorcluster)  [unwired: 2 in, 1 out]
                  n281 = GPIB Read(0:w328, 1:400, 3:w334) -> (5:w329:string, 7:w332:errorcluster)  [unwired: 2 in, 1 out]
                  n282 = local write "PI Stage Error 2"(w332) -> ()
                  n283 = Fract/Exp String To Number(string=w329) -> (number=w335:dbl)  [unwired: 3 in, 1 out]
                }
                n284 = call-poly <vilib>:"Mean.vi"("X"=w326) -> ("mean"=w325:dbl)  [unwired: 1 out]
                n285 = local read "Sensitivity Compensation"() -> (w324:dbl)
                n286 = Multiply(x=w325, y=w324) -> (x*y=w323:dbl)
                "Lockin realtime output" <- w323
                n287 = local write "Current Mean"(w323) -> ()
              }
            }
            n288 = Absolute Value(x=w201) -> (abs(x)=w200:dbl)
            n289 = Less Or Equal?(x=w200, y=0.1) -> (x <= y?=w203:bool)
            n290 = And(x=w203, y="Left jog") -> (x .and. y?=w202:bool)
            n291 = case shown="True" w202 {
              tunnel: w191 -> [_ w369]
              frame False {
              }
              frame True {
                n292 = flat-sequence {
                  tunnel: [w373] -> w371
                  tunnel: w369 -> [_]
                  tunnel: w371 -> [w379]
                  tunnel: [w378] -> w370
                  tunnel: [w376] -> w368
                  tunnel: w370 -> [w382]
                  tunnel: w368 -> [w383]
                  frame #0 {
                    n293 = local read "Stage Position"() -> (w372:dbl)
                    n294 = local read "PI Stage Error 2"() -> (w375:errorcluster)
                    n295 = call "movePI.vi"("PI Stage Error"=w375, "move to position"=w372) -> ("final position"=w374:dbl, "PI Stage Error 2"=w373:errorcluster)
                    n296 = local write "Stage Position"(w374) -> ()
                  }
                  frame #1 {
                    n297 = local read "Jog step size (mm)"() -> (w381:dbl)
                    n298 = local read "Stage Position"() -> (w380:dbl)
                    n299 = Subtract(x=w380, y=w381) -> (x-y=w377:dbl)
                    n300 = call "movePI.vi"("PI Stage Error"=w379, "move to position"=w377) -> ("final position"=w376:dbl, "PI Stage Error 2"=w378:errorcluster)
                  }
                  frame #2 {
                    n301 = local write "Stage Position"(w383) -> ()
                    n302 = local write "PI Stage Error 2"(w382) -> ()
                  }
                  frame #3 {
                    n303 = local write "Left jog"(FALSE) -> ()
                  }
                }
              }
            }
            n304 = local read "Jog step size (mm)"() -> (w194:dbl)
            n305 = Absolute Value(x=w194) -> (abs(x)=w193:dbl)
            n306 = Less Or Equal?(x=w193, y=0.1) -> (x <= y?=w198:bool)
            n307 = And(x=w198, y="Right jog") -> (x .and. y?=w197:bool)
            n308 = case shown="True" "Move to Position Button" {
              tunnel: w191 -> [_ w338]
              frame False {
              }
              frame True {
                n309 = flat-sequence {
                  tunnel: [w342] -> w339
                  tunnel: w338 -> [_]
                  tunnel: [w341] -> w336
                  tunnel: [w346] -> w340
                  tunnel: w339 -> [w346]
                  tunnel: [w345] -> w337
                  tunnel: w336 -> [w345]
                  tunnel: w340 -> [w348]
                  tunnel: w337 -> [w349]
                  frame #0 {
                    n310 = local read "PI Stage Error 2"() -> (w343:errorcluster)
                    n311 = local read "Position"() -> (w344:dbl)
                    n312 = call "movePI.vi"("PI Stage Error"=w343, "move to position"=w344) -> ("final position"=w341:dbl, "PI Stage Error 2"=w342:errorcluster)
                  }
                  frame #1 {
                    n313 = Wait (ms)(milliseconds to wait=200) -> ()  [unwired: 1 out]
                  }
                  frame #2 {
                    n314 = local write "PI Stage Error 2"(w348) -> ()
                    n315 = local write "Stage Position"(w349) -> ()
                  }
                  frame #3 {
                    n316 = local write "Move to Position Button"(FALSE) -> ()
                  }
                }
              }
            }
            n317 = case shown="True" w197 {
              tunnel: w191 -> [_ w353]
              frame False {
              }
              frame True {
                n318 = flat-sequence {
                  tunnel: w353 -> [_]
                  tunnel: [w355] -> w352
                  tunnel: [w360] -> w354
                  tunnel: w352 -> [w361]
                  tunnel: [w359] -> w351
                  tunnel: w354 -> [w365]
                  tunnel: w351 -> [w366]
                  frame #0 {
                    n319 = local read "Stage Position"() -> (w356:dbl)
                    n320 = local read "PI Stage Error 2"() -> (w357:errorcluster)
                    n321 = call "movePI.vi"("PI Stage Error"=w357, "move to position"=w356) -> ("final position"=w358:dbl, "PI Stage Error 2"=w355:errorcluster)
                    n322 = local write "Stage Position"(w358) -> ()
                  }
                  frame #1 {
                    n323 = local read "Jog step size (mm)"() -> (w364:dbl)
                    n324 = local read "Stage Position"() -> (w363:dbl)
                    n325 = Add(x=w363, y=w364) -> (x+y=w362:dbl)
                    n326 = call "movePI.vi"("PI Stage Error"=w361, "move to position"=w362) -> ("final position"=w359:dbl, "PI Stage Error 2"=w360:errorcluster)
                  }
                  frame #2 {
                    n327 = local write "Stage Position"(w366) -> ()
                    n328 = local write "PI Stage Error 2"(w365) -> ()
                  }
                  frame #3 {
                    n329 = local write "Right jog"(FALSE) -> ()
                  }
                }
              }
            }
            n330 = case shown="True" "Autophase" {
              frame False {
              }
              frame True {
                n331 = flat-sequence {
                  frame #0 {
                    n332 = local read "Lockin GPIB Address"() -> (w206:string)
                    n333 = local read "Lockin error out"() -> (w208:errorcluster)
                    n334 = GPIB Write(0:w206, 1:"APHS\n", 3:w208) -> (6:w207:errorcluster)  [unwired: 2 in, 1 out]
                    n335 = local write "Lockin error out"(w207) -> ()
                  }
                  frame #1 {
                    n336 = local write "Autophase"(FALSE) -> ()
                  }
                }
              }
            }
          }
        }
      }
    }
    frame #3 {
      n337 = local read "PI Stage Error 2"() -> (w387:errorcluster)
      n338 = call "Close connection if open.vi"("System no."=1, "error in"=w387) -> ("error out"=w386:errorcluster)  [unwired: 16 in, 1 out]
      n339 = local write "PI Stage Error 2"(w386) -> ()
    }
  }
